vi "GetDataTypeDescription.vi"(8 "error in (no error)":errorcluster, 11 "Value":variant) -> (0 "error out":errorcluster, 3 "Datatype Description":string)   [LabVIEW 2020, in "ContextHelpEditor.lvlib"]
uses:
  ContextHelpEditor.lvlib
  <vilib>/Utility/Data Type/NI_Data Type.lvlib
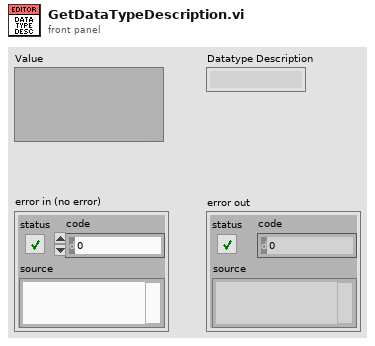
[diagram p1: front panel]
types:
  T1 = typedef "NI_Data Type.lvlib/Data Type.ctl" = enum8{"Invalid Type", "Void", "I8", "I16", "I32", "I64", "U8", "U16", "U32", "U64", "Single Float", "Double Float", "Extended Float", "Single Complex", "Double Complex", "Extended Complex", "Enum U8", "Enum U16", "Enum U32", "Enum U64", "Single Float With Unit", "Double Float With Unit", "Extended Float With Unit", "Single Complex with Unit", "Double Complex with Unit", "Extended Complex with Unit", "Boolean", "String", "Path", "Picture", "Tag", "Array", "Cluster", "Variant", "LV Variant", "Waveform", "Timestamp", "Digital Waveform", "Digital Data", "ExpressData", "Refnum", "External Data", "VI", "Poly VI", "LabVIEW Class Instance", "Fixed Point", "Set Collection", "Map Collection"}
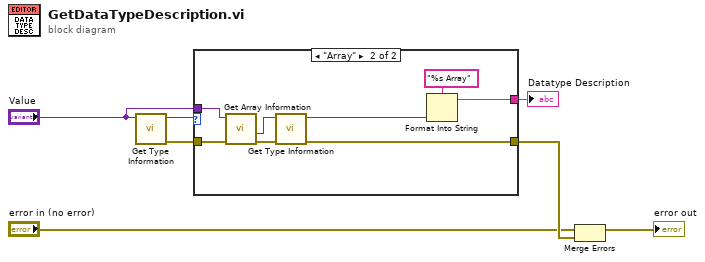
[diagram p0: block diagram]
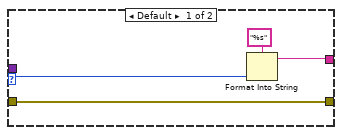
[diagram p2: hidden frame]
diagram:
  n1 = call <vilib>:"Get Type Information.vi"("variant"="Value") -> ("error out"=w4:errorcluster, "type"=w6:T1)  [unwired: 6 in, 3 out]
  n2 = case shown="\"Array\"" w6 {
    selector: w6 -> [w10 _]
    tunnel: w4 -> [w8 w19]
    tunnel: [w8 w15] -> w5
    tunnel: "Value" -> [_ w18]
    tunnel: [w11 w13] -> w1
    frame Default {
      n3 = Format Into String(format string="%s", w10) -> (resulting string=w11:string)  [unwired: 2 in, 1 out]
    }
    frame "Array" {
      n4 = call <vilib>:"Get Array Information.vi"("error in (no error)"=w19, "variant"=w18) -> ("error out"=w17:errorcluster, "array element data type"=w16:variant)  [unwired: 6 in, 2 out]
      n5 = call <vilib>:"Get Type Information.vi"("error in (no error)"=w17, "variant"=w16) -> ("error out"=w15:errorcluster, "type"=w14:T1)  [unwired: 5 in, 3 out]
      n6 = Format Into String(format string="%s Array", w14) -> (resulting string=w13:string)  [unwired: 2 in, 1 out]
    }
  }
  "Datatype Description" <- w1
  n7 = Merge Errors("error in (no error)", w5) -> (→"error out":errorcluster)
